vi "GetDatatype__slk_mt.vi"(8 "error in (no error)":errorcluster, 11 "case model in":refnum<class "CaseModel__slk_mt.lvclass">) -> (0 "error out":errorcluster, 2 "data type":u8, 3 "case model out":refnum<class "CaseModel__slk_mt.lvclass">)   [LabVIEW 2013, in "Lazyboots Menu Tool.lvlib" / "CaseModel__slk_mt.lvclass"]
doc: "Returns datatype of case model object."
uses:
  CaseModel__slk_mt.lvclass
panel:
  # "GetDatatype__slk_mt.vi\nReturns datatype of case model object.\n\nNOTICE -- YOU MUST LEAVE THIS NOTICE IN PLACE.\n\nCopyright (c) 2011, LIANG LIU Shawn.Liu.cn@gmail.com\nAll rights reserved.\n\nRedistribution and use in source and binary forms, with or without modification, are permitted provided that the following conditions are met:\n-Redistributions of source code must retain the above copyright notice, this list of conditions and the following disclaimer.\n-Redistributions in binary form must reproduce the above copyright notice, this list of conditions and the following disclaimer in the documentation and/or other materials provided with the distribution.\n-Neither the name of the eLp nor the names of its contributors may be used to endorse or promote products derived from this software without specific prior written permission.\n\nTHIS SOFTWARE IS PROVIDED BY THE COPYRIGHT HOLDERS AND CONTRIBUTORS \"AS IS\" AND ANY EXPRESS OR IMPLIED WARRANTIES, INCLUDING, BUT NOT LIMITED TO, THE IMPLIED WARRANTIES OF MERCHANTABILITY AND FITNESS FOR A PARTICULAR PURPOSE ARE DISCLAIMED. IN NO EVENT SHALL THE COPYRIGHT HOLDER OR CONTRIBUTORS BE LIABLE FOR ANY DIRECT, INDIRECT, INCIDENTAL, SPECIAL, EXEMPLARY, OR CONSEQUENTIAL DAMAGES (INCLUDING, BUT NOT LIMITED TO, PROCUREMENT OF SUBSTITUTE GOODS OR SERVICES; LOSS OF USE, DATA, OR PROFITS; OR BUSINESS INTERRUPTION) HOWEVER CAUSED AND ON ANY THEORY OF LIABILITY, WHETHER IN CONTRACT, STRICT LIABILITY, OR TORT (INCLUDING NEGLIGENCE OR OTHERWISE) ARISING IN ANY WAY OUT OF THE USE OF THIS SOFTWARE, EVEN IF ADVISED OF THE POSSIBILITY OF SUCH DAMAGE."
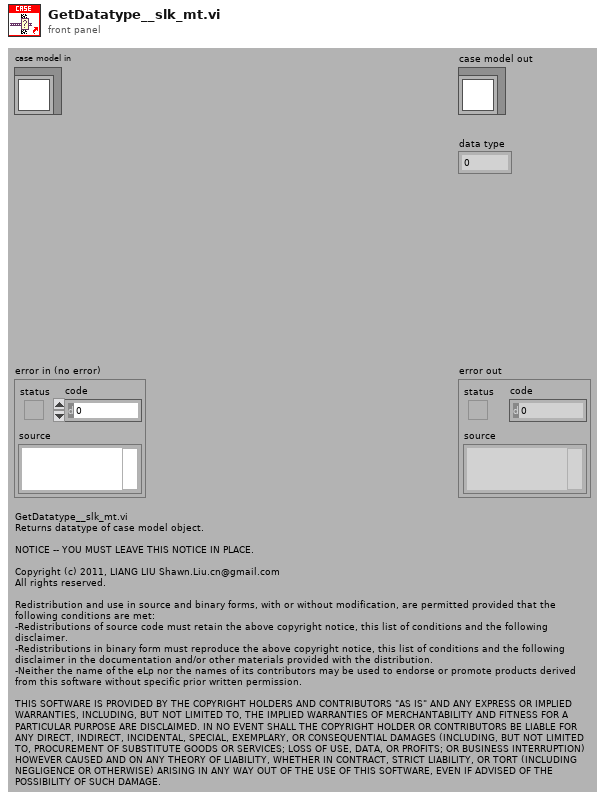
[diagram p1: front panel]
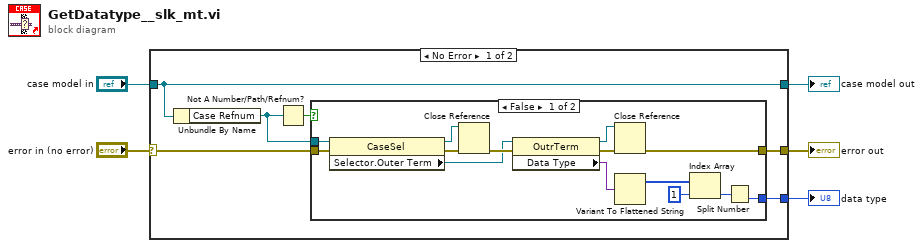
[diagram p0: block diagram]
diagram:
  n1 = case shown="No Error" "error in (no error)" {
    selector: "error in (no error)" -> [w9 w27]
    tunnel: [w8 w27] -> w4
    tunnel: [w11 w28] -> w2
    tunnel: "case model in" -> [w11 w28]
    tunnel: [w10 _] -> w1
    frame No Error {
      n2 = Unbundle By Name(w11) -> ("Case Refnum"=w6:refnum<vi>)
      n3 = Not A Number/Path/Refnum?(number/path/refnum=w6) -> (NaN/Path/Refnum?=w7:bool)
      n4 = case shown="False" w7 {
        tunnel: w6 -> [w17 _]
        tunnel: [w16 _] -> w10
        tunnel: w9 -> [w15 w26]
        tunnel: [w13 w26] -> w8
        frame False {
          n5 = property class="CaseSel"(reference=w17, error in=w15) -> (reference out=w21:refnum<vi>, error out=w19:errorcluster, "Selector.Outer Term"=w18:refnum<vi>)
          n6 = Close Reference(reference=w21, error in (no error)=w19) -> (error out=w20:errorcluster)
          n7 = property class="OutrTerm"(reference=w18, error in=w20) -> (reference out=w12:refnum<vi>, error out=w14:errorcluster, "Data Type"=w22:variant)
          n8 = Close Reference(reference=w12, error in (no error)=w14) -> (error out=w13:errorcluster)
          n9 = Variant To Flattened String(Variant=w22) -> (1:w23:i16[])  [unwired: 1 out]
          n10 = Index Array(array=w23, index=1) -> (element=w25:i16)
          n11 = Split Number(x=w25) -> (lo(x)=w16:u8)  [unwired: 1 out]
        }
        frame True {
        }
      }
    }
    frame Error {
    }
  }
  "error out" <- w4
  "case model out" <- w2
  "data type" <- w1
